vi "Errors.vi"(8 "error in":errorcluster, 10 "Enum":T1(ring), 11 "JSON-RPC in":refnum<class "JSON-RPC.lvclass">) -> (0 "error out":errorcluster, 3 "JSON-RPC out":refnum<class "JSON-RPC.lvclass">)   [LabVIEW 2019, in "JSON-RPC.lvclass"]
uses:
  JSON-RPC.lvclass
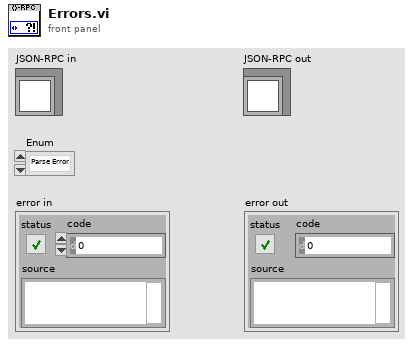
[diagram p1: front panel]
types:
  T1 = enum16{"Parse Error", "Invalid Request", "Method not found", "Invalid params", "Internal error", "Server error"}
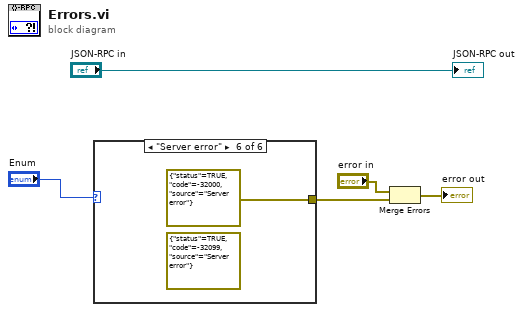
[diagram p0: block diagram]
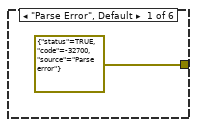
[diagram p2: hidden frame]
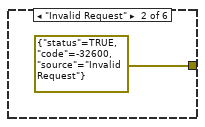
[diagram p3: hidden frame]
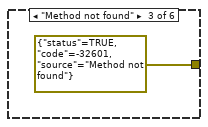
[diagram p4: hidden frame]
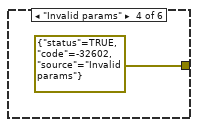
[diagram p5: hidden frame]
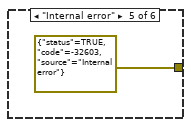
[diagram p6: hidden frame]
diagram:
  n1 = case shown="\"Server error\"" "Enum" {
    tunnel: [errorcluster {"status"=TRUE, "code"=-32700, "source"="Parse error"} ("error out") errorcluster {"status"=TRUE, "code"=-32600, "source"="Invalid Request"} ("error out") errorcluster {"status"=TRUE, "code"=-32601, "source"="Method not found"} ("error out") errorcluster {"status"=TRUE, "code"=-32602, "source"="Invalid params"} ("error out") errorcluster {"status"=TRUE, "code"=-32603, "source"="Internal error"} ("error out") errorcluster {"status"=TRUE, "code"=-32000, "source"="Server error"} ("error out")] -> w3
    frame "Parse Error", Default {
    }
    frame "Invalid Request" {
    }
    frame "Method not found" {
    }
    frame "Invalid params" {
    }
    frame "Internal error" {
    }
    frame "Server error" {
      (unwired) errorcluster {"status"=TRUE, "code"=-32099, "source"="Server error"} ("error out")
    }
  }
  n2 = Merge Errors("error in", w3) -> (→"error out":errorcluster)
  "JSON-RPC out" <- "JSON-RPC in"
